vi "Renew Search Result From Database.vi"(8 "error in (no error)":errorcluster, 10 "Keyword(\"\")":string, 11 "ToolLauncher in":refnum<class "ScriptDialog.lvclass">) -> (0 "error out":errorcluster, 3 "ToolLauncher out":refnum<class "ScriptDialog.lvclass">)   [LabVIEW 2015, in "ScriptDialog.lvclass"]
uses:
  <vilib>/LazyBootMenu/ToolLauncher/ScriptDialog.lvclass
  <vilib>/LazyBootMenu/ToolLauncher/ScriptDialog.lvclass/ScriptDialog.ctl
  <vilib>/LazyBootMenu/QDSearchList/QDDialogList.lvclass
  <vilib>/LazyBootMenu/_Database/Implements/ScriptDatabase.lvclass
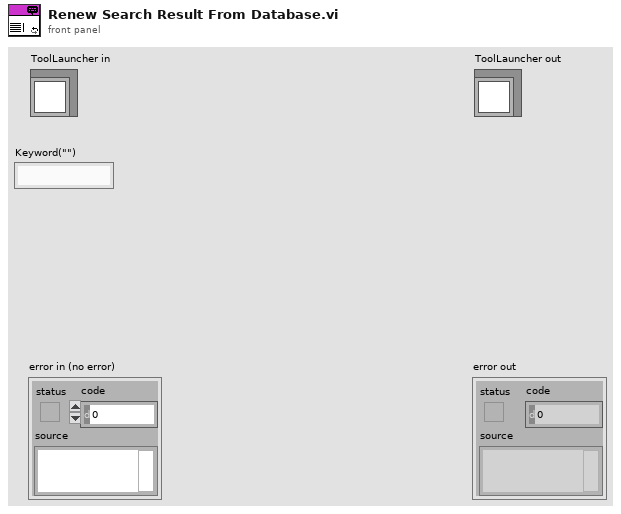
[diagram p1: front panel]
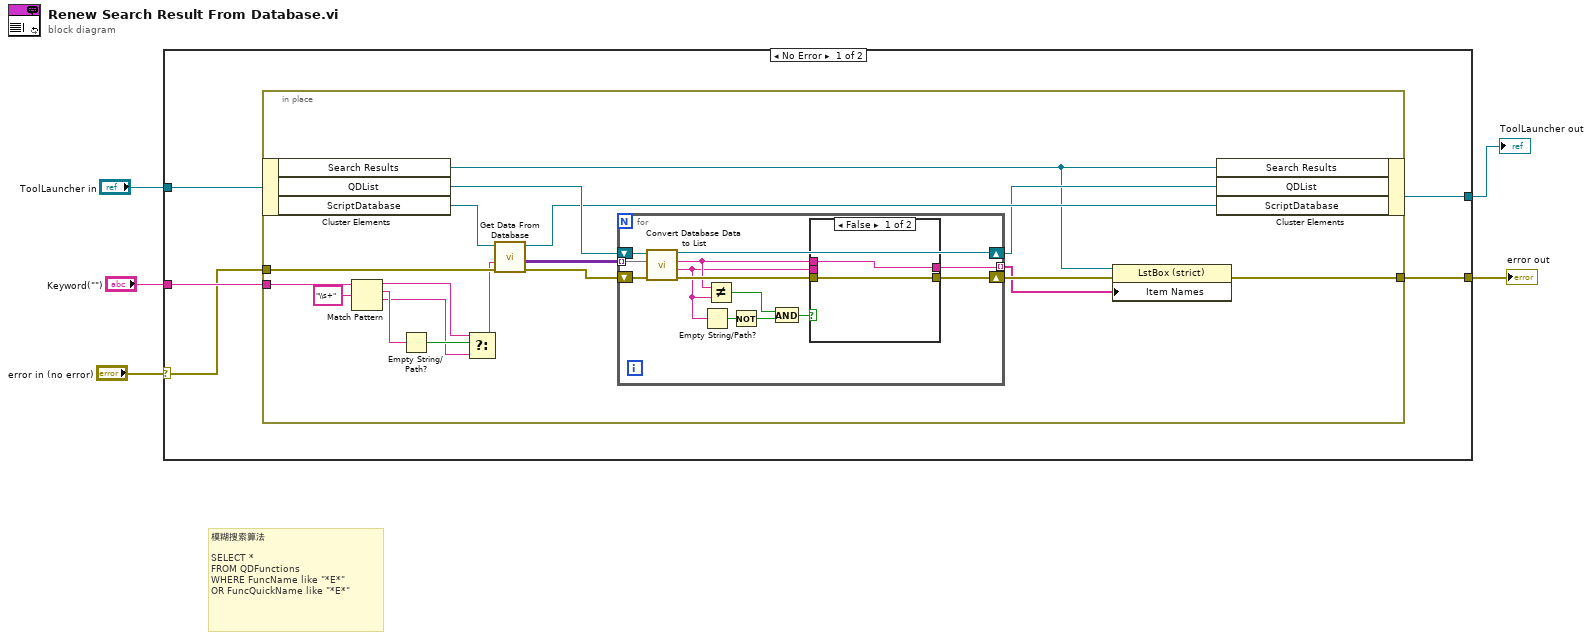
[diagram p0: block diagram]
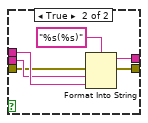
[diagram p2: hidden frame]
diagram:
  # "模糊搜索算法\n\nSELECT *\nFROM QDFunctions\nWHERE FuncName like \"*E*\" \nOR FuncQuickName like \"*E*\""
  n1 = case shown="No Error" "error in (no error)" {
    selector: "error in (no error)" -> [w8 w51]
    tunnel: "ToolLauncher in" -> [w10 w50]
    tunnel: "Keyword(\"\")" -> [w9 _]
    tunnel: [w6 w51] -> w2
    tunnel: [w7 w50] -> w1
    frame No Error {
      n2 = in-place "In Place Element Structure" {
        in-place-border: w9 -> [w17]
        in-place-border: w8 -> [w28]
        in-place-border: [w20] -> w6
        n3 = in-place-cluster #1(w10) -> ("Search Results"=w19:refnum<vi>, "QDList"=w24:refnum<class "QDDialogList.lvclass">, "ScriptDatabase"=w25:refnum<class "ScriptDatabase.lvclass">)
        n4 = Match Pattern(string=w17, regular expression="\\s+") -> (before substring=w13:string, match substring=w15:string, after substring=w12:string)  [unwired: 1 in, 1 out]
        n5 = Empty String/Path?(string/path=w15) -> (empty?=w14:bool)
        n6 = Select(t=w13, s=w14, f=w12) -> (s? t:f=w11:string)
        n7 = call <vilib>:"Get Data From Database.vi"("error in (no error)"=w28, "Keyword(\"\")"=w11, "ScriptDatabase in"=w25) -> ("error out"=w26:errorcluster, "recordset data"=w27:variant[][], "Database Out"=w23:refnum<class "ScriptDatabase.lvclass">)  [unwired: 6 in]
        n8 = for {
          tunnel: w27 -> [w41] mode=indexing
          shift-right: [w32] -> w21
          shift-left: w26 -> [w40]
          shift-right: [w33] -> w22
          shift-left: w24 -> [w39]
          tunnel: [w31] -> w18 mode=indexing
          n9 = call-dynamic "Convert Database Data to List.vi"("error in (no error)"=w40, "FetchedData"=w41, "NormalQDFunc in"=w39) -> ("error out"=w36:errorcluster, "QDFunction Acronym"=w34:string, "QDFunction Name"=w35:string, "NormalQDFunc out"=w33:refnum<class "QDDialogList.lvclass">)  [unwired: 5 in]
          n10 = Empty String/Path?(string/path=w34) -> (empty?=w30:bool)
          n11 = Not Equal?(x=w35, y=w34) -> (x != y?=w38:bool)
          n12 = Not(x=w30) -> (.not. x?=w29:bool)
          n13 = And(x=w38, y=w29) -> (x .and. y?=w37:bool)
          n14 = case shown="False" w37 {
            tunnel: w36 -> [w42 w45]
            tunnel: w35 -> [w43 w48]
            tunnel: w34 -> [_ w47]
            tunnel: [w43 w46] -> w31
            tunnel: [w42 w44] -> w32
            frame False {
            }
            frame True {
              n15 = Format Into String(format string="%s(%s)", error in=w45, w47, w48) -> (resulting string=w46:string, error out=w44:errorcluster)  [unwired: 1 in]
            }
          }
        }
        n16 = property class="LstBox (strict)"(reference=w19, error in=w21, "Item Names"=w18) -> (error out=w20:errorcluster)  [unwired: 1 out]
        n17 = in-place-cluster #1("Search Results"=w19, "QDList"=w22, "ScriptDatabase"=w23) -> (w7:refnum<class "ScriptDialog.lvclass">)
      }
    }
    frame Error {
    }
  }
  "error out" <- w2
  "ToolLauncher out" <- w1
